vi "select_camera.vi"() -> (0 "error out":errorcluster, 2 "Camera":T2, 3 "Session Out":T1="cam0", 4 "Session error":errorcluster={"status"=TRUE, "code"=-1, "source"="No session is open"})   [LabVIEW 2014]
uses:
  <vilib>/userdefined/High Color/IMAQdx.ctl
  <vilib>/vision/driver/IMAQdx.llb/IMAQdx Camera Control Mode.ctl
  <vilib>/vision/driver/NI_Vision_Acquisition_Software.lvlib
  <resource>/objmgr/imaqdx.rc
panel:
  in  "Listbox":i32(listbox)
  out "source":string
  out "OldVal":T1
  in  "Cancel Button":bool
  in  "Okay":bool
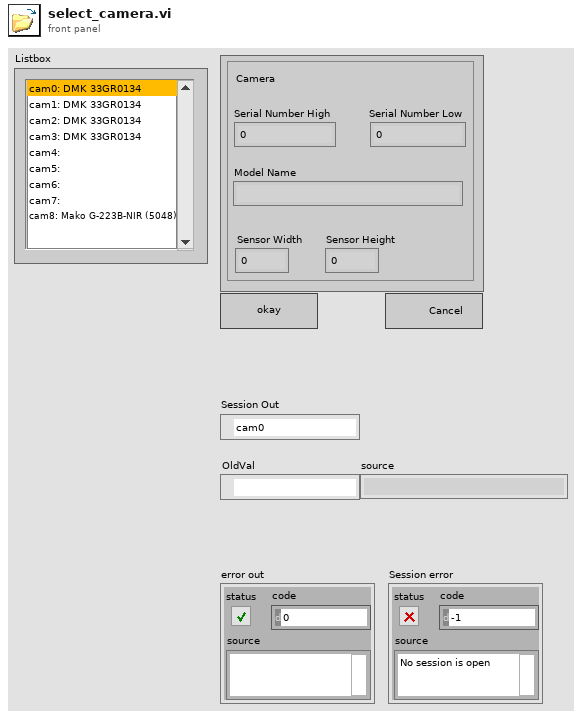
[diagram p1: front panel]
types:
  T1 = typedef "IMAQdx.ctl" = refnum<k21>
  T2 = cluster{"Serial Number High":u32, "Model Name":string, "Sensor Width":u32, "Sensor Height":u32, "Serial Number Low":u32}
  T3 = typedef "NI_Vision_Acquisition_Software.lvlib/IMAQdx Camera Control Mode.ctl" = enum16{"Controller", "Listener"}
  T4 = cluster{"Type":u32, "Version":u32, "Flags":u32, "SerialNumberHigh":u32, "SerialNumberLow":u32, "BusType":u32, "InterfaceName":string, "VendorName":string, "ModelName":string, "CameraFileName":string, "CameraAttributeURL":string}[]
  T5 = cluster{"SerialNumberHigh":u32, "ModelName":string, "Width":u32, "Height":u32, "SerialNumberLow":u32}
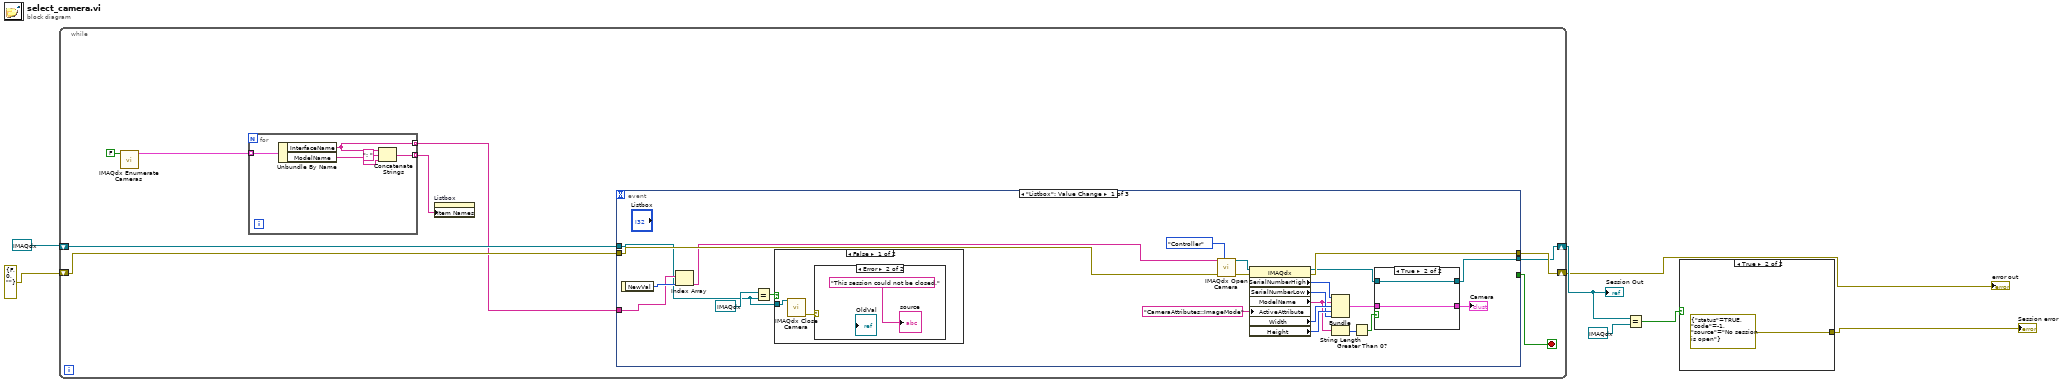
[diagram p0: block diagram]
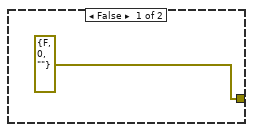
[diagram p2: hidden frame]
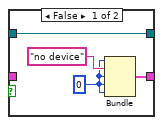
[diagram p3: hidden frame]
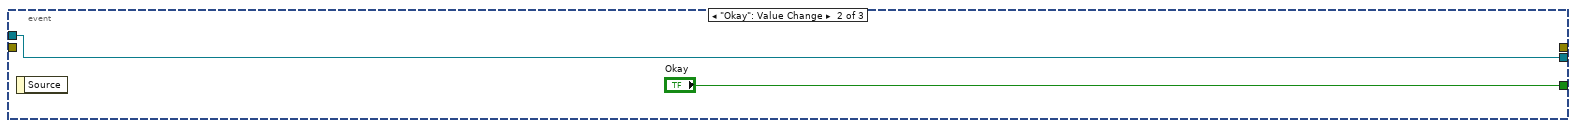
[diagram p6: hidden frame]
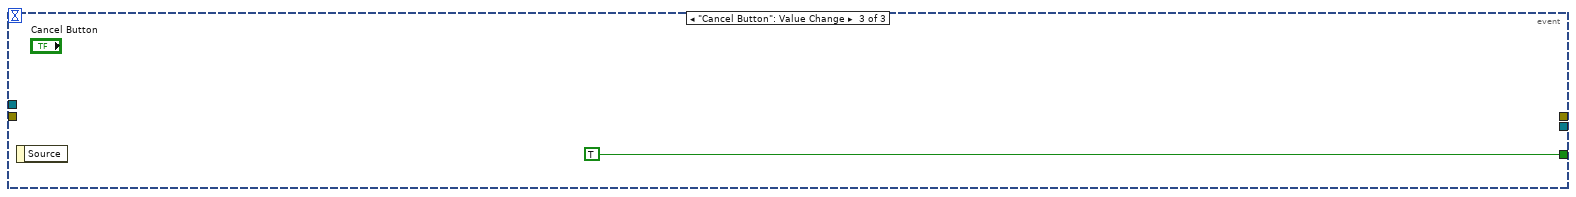
[diagram p7: hidden frame]
diagram:
  n1 = while {
    shift-right: [w16] -> w1
    shift-left: errorcluster {"status"=FALSE, "code"=0, "source"=""} ("error out") -> [w12]
    shift-right: [w15] -> w5
    shift-left: T1 refnum ("Session Out 2") -> [w14]
    stop <- w13 stop-if-true
    n2 = call <vilib>:"IMAQdx Enumerate Cameras.vi"("Connected Only? (Yes)"=FALSE) -> ("Camera Information Array"=w10:T4)  [unwired: 9 in, 1 out]
    n3 = for {
      tunnel: w10 -> [w21] mode=indexing
      tunnel: [w18] -> w9 mode=indexing
      tunnel: [w17] -> w8 mode=indexing
      n4 = Unbundle By Name(w21) -> ("InterfaceName"=w17:string, "ModelName"=w19:string)
      n5 = Concatenate Strings(w17, ": " ("string"), w19) -> (w18:string)
    }
    n6 = property on="Listbox" class="LstBox (strict)"("Item Names"=w9) -> ()  [unwired: 2 in, 2 out]
    n7 = event shown="[0] \"Listbox\": Value Change" {
      selector: _ -> [_ _ _]
      dyn-events: _ -> [_ _ _]
      timeout: _ -> [_ _ _]
      tunnel: [w44 _ _] -> w16
      tunnel: [_ "Okay" TRUE] -> w13
      tunnel: [w43 w54 _] -> w15
      tunnel: w14 -> [w22 w54 _]
      tunnel: w12 -> [w42 _ _]
      tunnel: w8 -> [w24 _ _]
      event "Listbox": Value Change {
        n8 = event-data() -> ("NewVal"=w25:i32)  [unwired: 1 in]
        n9 = Index Array(array=w24, index=w25) -> (element=w23:string)
        n10 = Equal?(x=T1 refnum ("Session Out 2"), y=w22) -> (x = y?=w40:bool)
        n11 = case shown="False" w40 {
          tunnel: w22 -> [w51 _]
          frame False {
            n12 = call <vilib>:"IMAQdx Close Camera.vi"("Session In"=w51) -> ("error out"=w52:errorcluster)  [unwired: 10 in]
            n13 = case shown="Error" w52 {
              frame No Error {
              }
              frame Error {
                "source" <- "This session could not be closed." ("source")
              }
            }
          }
          frame True {
          }
        }
        n14 = call <vilib>:"IMAQdx Open Camera.vi"("Camera Control Mode"=IMAQdx_Camera_Control_Mode."Controller", "error in"=w42, "Session In"=w23) -> ("error out"=w28:errorcluster, "Session Out"=w29:T1)  [unwired: 7 in]
        n15 = property class="IMAQdx"(reference=w29, error in=w28, "ActiveAttribute"="CameraAttributes::ImageMode") -> (reference out=w30:T1, error out=w44:errorcluster, "SerialNumberHigh"=w39:u32, "SerialNumberLow"=w33:u32, "ModelName"=w32:string, "Width"=w35:u32, "Height"=w34:u32)
        n16 = Bundle("SerialNumberHigh"=w39, "ModelName"=w32, "Width"=w35, "Height"=w34, "SerialNumberLow"=w33) -> (w36:T5)  [unwired: 1 in]
        n17 = String Length(string=w32) -> (length=w38:i32)
        n18 = Greater Than 0?(x=w38) -> (x > 0?=w37:bool)
        n19 = case shown="True" w37 {
          tunnel: [w45 w50] -> w43
          tunnel: w30 -> [w45 w50]
          tunnel: [w48 w49] -> w31
          tunnel: w36 -> [_ w49]
          frame False {
            w46 = 0
            n20 = Bundle(w46, "no device", w46, w46, w46) -> (w48:cluster{i32, string, i32, i32, i32})  [unwired: 1 in]
          }
          frame True {
          }
        }
        "Camera" <- w31
      }
      event "Okay": Value Change {
        n21 = event-data() -> ()  [unwired: 1 in, 1 out]
      }
      event "Cancel Button": Value Change {
        n22 = event-data() -> ()  [unwired: 1 in, 1 out]
      }
    }
  }
  "error out" <- w1
  "Session Out" <- w5
  n23 = Equal?(x=w5, y=T1 refnum ("Session Out 2")) -> (x = y?=w3:bool)
  n24 = case shown="True" w3 {
    tunnel: [errorcluster {"status"=FALSE, "code"=0, "source"=""} ("error out") errorcluster {"status"=TRUE, "code"=-1, "source"="No session is open"} ("error out")] -> w2
    frame False {
    }
    frame True {
    }
  }
  "Session error" <- w2
